vi "Read Config Version.vi"(8 "error in (no error)":errorcluster, 11 "System Config Server in":refnum<class "System Config Module.lvclass">) -> (0 "error out":errorcluster, 3 "System Config Server out":refnum<class "System Config Module.lvclass">)   [LabVIEW 2020, in "Volatus.lvlib" / "System Config Module.lvclass"]
uses:
  System Config Module.lvclass
  C:/dev/lv20CE/relink/lv-volatus/Volatus/Module/Module.lvclass
  VolatusConfig/Meta Name.ctl
  Module/Module.lvclass/Module.ctl
  VolatusConfig/VolatusConfigElement/VolatusConfigElement.lvclass/VolatusConfigElement.ctl
  System Config Module.lvclass/System Config Module.ctl
  VolatusConfig/VolatusConfigElement/Element.vi
  lv-cdm/CDM-Config/Config Element/Owner.vi
  Module/Module.lvclass
  VolatusConfig/VolatusConfigElement/VolatusConfigElement.lvclass
  lv-cdm/CDM-Config/Config Filter/Config Lookup.lvclass
  lv-cdm/CDM-Config/Config Element/Config Element.lvclass
  VolatusConfig/VolatusConfig.lvlib
  lv-builder/Builder Core/Builder Core.lvlib
  C:/dev/lv20CE/relink/lv-volatus/Volatus/System Config Server/System Config Module.lvclass
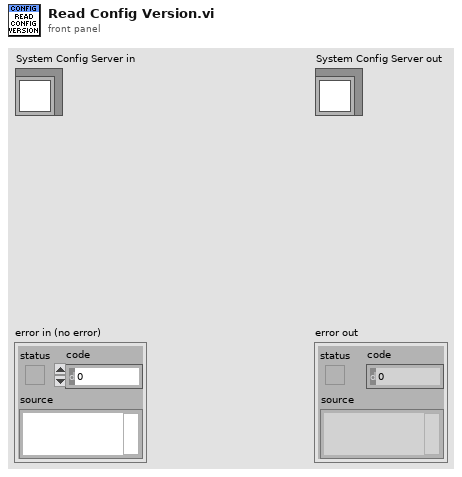
[diagram p1: front panel]
types:
  T1 = typedef "VolatusConfig.lvlib/Meta Name.ctl" = enum16{"VL_Type", "VL_Node_IP", "VL_Node_Type", "VL_Task_Type", "VL_Group_Type", "VL_Channel_Type", "VL_Channel_DataType", "VL_Config_Version", "VL_Overlay_Type"}
  T2 = typedef "Builder Core.lvlib/Version.ctl" = cluster{"Major":u16, "Minor":u16, "Fix":u16, "Build":u16}
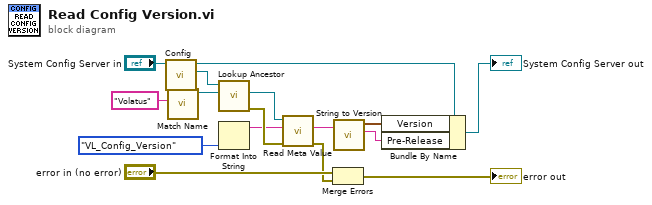
[diagram p0: block diagram]
diagram:
  n1 = call "Config.vi"("Module in"="System Config Server in") -> ("Config"=w15:refnum<class "VolatusConfigElement.lvclass">, "Module out"=w7:refnum<class "System Config Module.lvclass">)  [unwired: 9 in]
  n2 = call "Match Name.vi"("Name"="Volatus") -> ("Config Lookup out"=w14:refnum<class "Config Lookup.lvclass">)  [unwired: 9 in, 1 out]
  n3 = call "Lookup Ancestor.vi"("Lookup"=w14, "VolatusConfigElement in"=w15) -> ("error out"=w16:errorcluster, "Ancestor"=w12:refnum<class "Config Element.lvclass">)  [unwired: 7 in, 1 out]
  n4 = Format Into String(Meta_Name."VL_Config_Version" ("Meta Name")) -> (resulting string=w10:string)  [unwired: 3 in, 1 out]
  n5 = call "Read Meta Value.vi"("error in (no error)"=w16, "Meta Name"=w10, "Config Element in"=w12) -> ("error out"=w2:errorcluster, "Meta Value"=w9:string)  [unwired: 6 in, 1 out]
  n6 = Merge Errors("error in (no error)", w2) -> (→"error out":errorcluster)
  n7 = call "String to Version.vi"("Version String"=w9) -> ("Version"=w5:T2, "Pre-Release"=w4:string)  [unwired: 4 in, 1 out]
  n8 = Bundle By Name(cluster=w7, "Version"=w5, "Pre-Release"=w4) -> (→"System Config Server out":refnum<class "System Config Module.lvclass">)
